vi "WriteData.vi"(8 "error in (no error)":errorcluster, 10 "Data":string, 11 "Connection in":refnum<class "Connection.lvclass">) -> (0 "error out":errorcluster, 3 "Connection out":refnum<class "Connection.lvclass">)   [LabVIEW 2022 SP3, in "Connection.lvlib" / "Connection.lvclass"]
uses:
  Connection.lvclass
  Connection.lvclass/Connection.ctl
  TcpSocket/Source/TcpSocket/Connection/Connection.lvclass
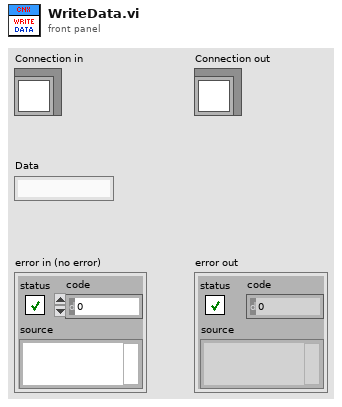
[diagram p1: front panel]
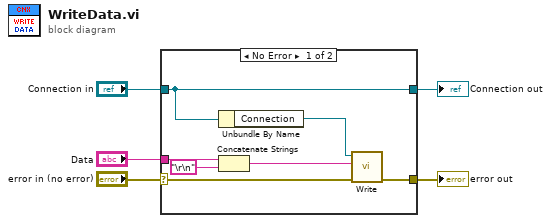
[diagram p0: block diagram]
diagram:
  n1 = case shown="No Error" "error in (no error)" {
    selector: "error in (no error)" -> [w11 w14]
    tunnel: [w10 w14] -> w4
    tunnel: [w12 w13] -> w2
    tunnel: "Connection in" -> [w12 w13]
    tunnel: "Data" -> [w7 _]
    frame No Error {
      n2 = Unbundle By Name(w12) -> ("Connection"=w6:refnum<class "Connection.lvclass">)
      n3 = Concatenate Strings(w7, "\r\n") -> (w8:string)
      n4 = call-dynamic "Write.vi"("error in (no error)"=w11, "Data"=w8, "Connection in"=w6) -> ("error out"=w10:errorcluster)  [unwired: 7 in, 1 out]
    }
    frame Error {
    }
  }
  "error out" <- w4
  "Connection out" <- w2
